vi "Write TCS parameters.vi"(8 "error in (no error)":errorcluster, 10 "TCS parameters":T1, 11 "TCS_ACS in":refnum<class "TCS_ACS.lvclass">) -> (0 "error out":errorcluster, 3 "TCS_ACS out":refnum<class "TCS_ACS.lvclass">)   [LabVIEW 2018, in "TCS_ACS.lvclass"]
uses:
  TCS_ACS.lvclass
  TCS_ACS.lvclass/TCS_ACS.ctl
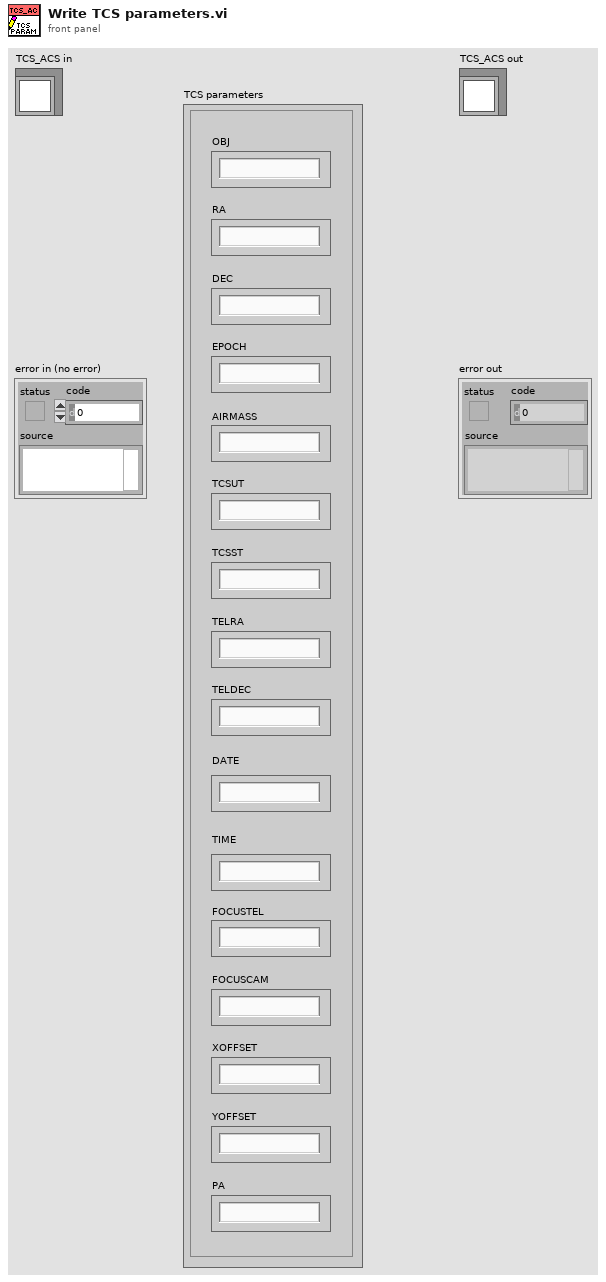
[diagram p1: front panel]
types:
  T1 = cluster{"OBJ":string, "RA":string, "DEC":string, "EPOCH":string, "AIRMASS":string, "TCSUT":string, "TCSST":string, "TELRA":string, "TELDEC":string, "DATE":string, "TIME":string, "FOCUSTEL":string, "FOCUSCAM":string, "XOFFSET":string, "YOFFSET":string, "PA":string}
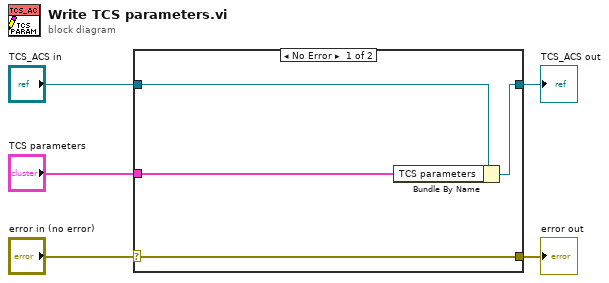
[diagram p0: block diagram]
diagram:
  n1 = case shown="No Error" "error in (no error)" {
    selector: "error in (no error)" -> [w9 w10]
    tunnel: [w9 w10] -> w4
    tunnel: [w7 w11] -> w2
    tunnel: "TCS_ACS in" -> [w8 w11]
    tunnel: "TCS parameters" -> [w6 _]
    frame No Error {
      n2 = Bundle By Name(cluster=w8, "TCS parameters"=w6) -> (w7:refnum<class "TCS_ACS.lvclass">)
    }
    frame Error {
    }
  }
  "error out" <- w4
  "TCS_ACS out" <- w2
